vi "MindwaveGetPLENGTH.vi"(3 "error in (no error) input":errorcluster, 5 "VISA resource name input":refnum<visa-resource-name>) -> (0 "error out":errorcluster, 1 "[PLENGTH]":u8 format="%x", 2 "VISA resource name out":refnum<visa-resource-name>)   [LabVIEW 2011, in "Neurosky.lvlib"]
uses:
  Users/Isaias/Documents/GitHub/Neurosky/Neurosky.lvlib
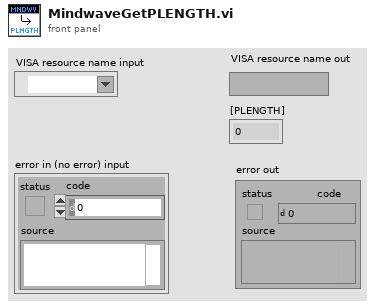
[diagram p1: front panel]
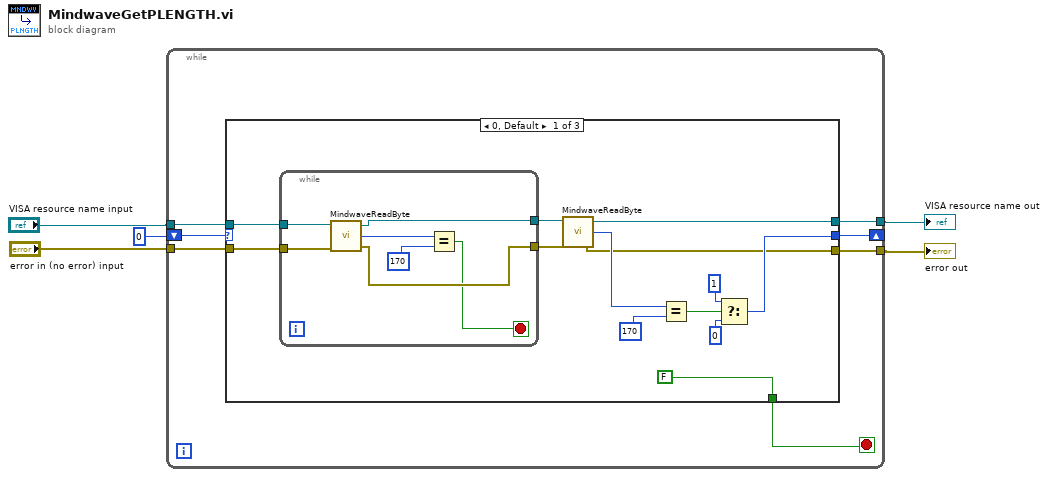
[diagram p0: block diagram]
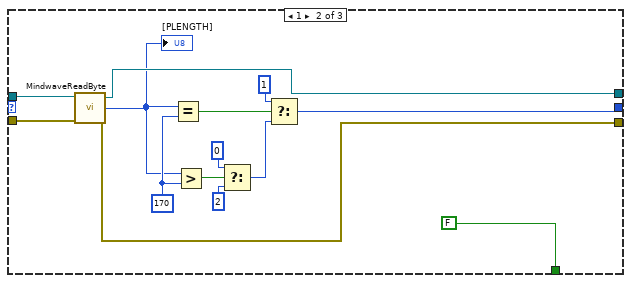
[diagram p2: hidden frame]
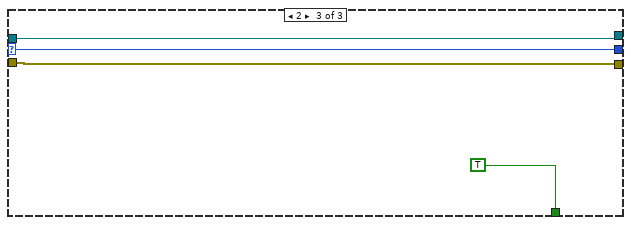
[diagram p3: hidden frame]
diagram:
  n1 = while {
    shift-right: [w12] -> _
    shift-left: u8 0 -> [w11]
    tunnel: [w10] -> w2
    tunnel: [w9] -> w1
    tunnel: "VISA resource name input" -> [w8]
    tunnel: "error in (no error) input" -> [w7]
    stop <- w6 stop-if-true
    n2 = case shown="0, Default" w11 {
      selector: w11 -> [_ _ w50]
      tunnel: [w20 w37 w50] -> w12
      tunnel: [w17 w44 w49] -> w9
      tunnel: [w14 w34 w48] -> w10
      tunnel: [FALSE FALSE TRUE] -> w6
      tunnel: w8 -> [w16 w36 w49]
      tunnel: w7 -> [w15 w35 w48]
      frame 0, Default {
        n3 = while {
          tunnel: [w30] -> w19
          tunnel: [w27] -> w18
          tunnel: w16 -> [w29]
          tunnel: w15 -> [w28]
          stop <- w26 stop-if-true
          n4 = call <userlib>:"MindwaveReadByte.vi"("error in (no error) input"=w28, "VISA resource name input"=w29) -> ("error out"=w27:errorcluster, "byte"=w31:u8, "VISA resource name out"=w30:refnum<visa-resource-name>)  [unwired: 2 in]
          n5 = Equal?(x=w31, y=u8 170) -> (x = y?=w26:bool)
        }
        n6 = call <userlib>:"MindwaveReadByte.vi"("error in (no error) input"=w18, "VISA resource name input"=w19) -> ("error out"=w14:errorcluster, "byte"=w24:u8, "VISA resource name out"=w17:refnum<visa-resource-name>)  [unwired: 2 in]
        n7 = Equal?(x=w24, y=u8 170) -> (x = y?=w23:bool)
        n8 = Select(t=u8 1, s=w23, f=u8 0) -> (s? t:f=w20:u8)
      }
      frame 1 {
        w43 = u8 170
        n9 = call <userlib>:"MindwaveReadByte.vi"("error in (no error) input"=w35, "VISA resource name input"=w36) -> ("error out"=w34:errorcluster, "byte"=w42:u8, "VISA resource name out"=w44:refnum<visa-resource-name>)  [unwired: 2 in]
        "[PLENGTH]" <- w42
        n10 = Equal?(x=w42, y=w43) -> (x = y?=w46:bool)
        n11 = Greater?(x=w42, y=w43) -> (0:w39:bool)
        n12 = Select(t=u8 0, s=w39, f=u8 2) -> (s? t:f=w38:u8)
        n13 = Select(t=u8 1, s=w46, f=w38) -> (s? t:f=w37:u8)
      }
      frame 2 {
      }
    }
  }
  "VISA resource name out" <- w1
  "error out" <- w2
